vi "Get Trigger Timer Count.vi"(8 "error in (no error)":errorcluster, 10 "Timer (1)":i32=1 format="%#.6g", 11 "VISA resource name":refnum<visa-resource-name>) -> (0 "error out":errorcluster, 2 "Count":dbl, 3 "VISA resource name out":refnum<visa-resource-name>)   [LabVIEW 2020, in "Keithley 2450.lvlib"]
doc: "Gets the number of events to generate each time the timer detects its trigger event or is enabled as a timer or alarm"
uses:
  <instrlib>/Keithley 2450/Keithley 2450.lvlib
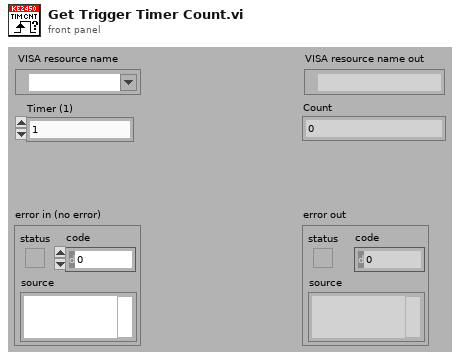
[diagram p1: front panel]
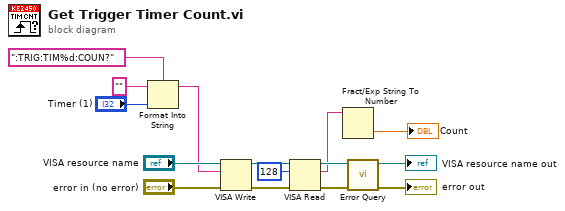
[diagram p0: block diagram]
diagram:
  n1 = Format Into String(format string=":TRIG:TIM%d:COUN?", initial string="", "Timer (1)") -> (resulting string=w8:string)  [unwired: 1 in, 1 out]
  n2 = VISA Write(VISA resource name="VISA resource name", write buffer=w8, error in (no error)="error in (no error)") -> (VISA resource name out=w5:refnum<visa-resource-name>, error out=w7:errorcluster)  [unwired: 1 out]
  n3 = VISA Read(VISA resource name=w5, byte count=u32 128, error in (no error)=w7) -> (VISA resource name out=w4:refnum<visa-resource-name>, read buffer=w2:string, error out=w6:errorcluster)  [unwired: 1 out]
  n4 = Fract/Exp String To Number(string=w2) -> (number=→"Count":dbl)  [unwired: 3 in, 1 out]
  n5 = call <instrlib>:"Error Query.vi"("error in (no error)"=w6, "VISA resource name"=w4) -> ("error out"=→"error out":errorcluster, "VISA resource name out"=→"VISA resource name out":refnum<visa-resource-name>)  [unwired: 8 out]
